vi "CloseNotifier.vi"(8 "entrée d'erreur":errorcluster caption="entrée d'erreur (pas d'erreur)", 11 "Notifiers":T1) -> (0 "error out":errorcluster)   [LabVIEW 2017, in "Notifier.lvlib"]
doc: "Ce VI permet la suppression de tous les notifiers à la fin de l'utilisation du centre d'usinage. Doit être modifier si un appareil a été ajouté ou supprimé."
uses:
  Notifier.lvlib
  Notifier.ctl
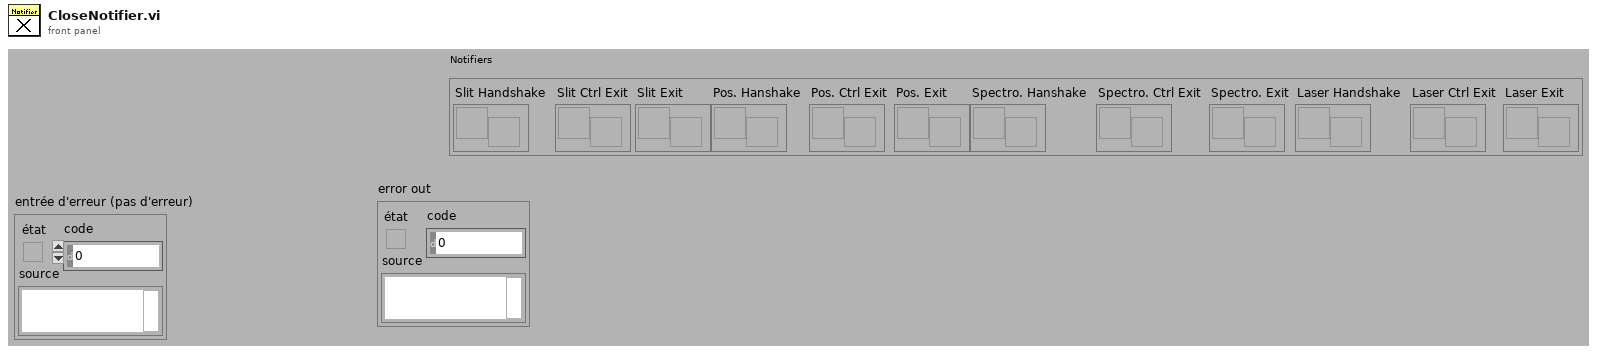
[diagram p1: front panel]
types:
  T1 = typedef "Notifier.lvlib/Notifier.ctl" = cluster{"Slit Handshake":refnum<notifier>, "Slit Ctrl Exit":refnum<notifier>, "Slit Exit":refnum<notifier>, "Pos. Hanshake":refnum<notifier>, "Pos. Ctrl Exit":refnum<notifier>, "Pos. Exit":refnum<notifier>, "Spectro. Hanshake":refnum<notifier>, "Spectro. Ctrl Exit":refnum<notifier>, "Spectro. Exit":refnum<notifier>, "Laser Handshake":refnum<notifier>, "Laser Ctrl Exit":refnum<notifier>, "Laser Exit":refnum<notifier>}
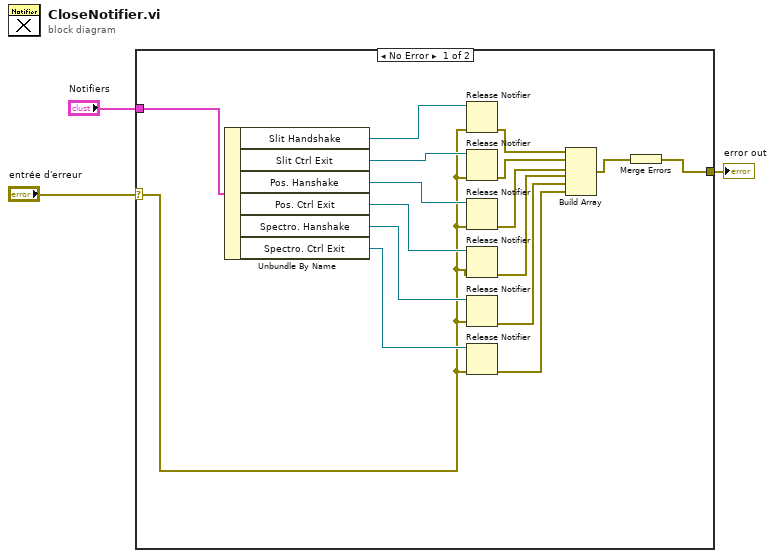
[diagram p0: block diagram]
diagram:
  n1 = case shown="No Error" "entrée d'erreur" {
    selector: "entrée d'erreur" -> [w4 w20]
    tunnel: "Notifiers" -> [w19 _]
    tunnel: [w11 w20] -> w1
    frame No Error {
      n2 = Unbundle By Name(w19) -> ("Slit Handshake"=w18:refnum<notifier>, "Slit Ctrl Exit"=w17:refnum<notifier>, "Pos. Hanshake"=w16:refnum<notifier>, "Pos. Ctrl Exit"=w10:refnum<notifier>, "Spectro. Hanshake"=w9:refnum<notifier>, "Spectro. Ctrl Exit"=w8:refnum<notifier>)
      n3 = Release Notifier(notifier=w18, error in (no error)=w4) -> (error out=w15:errorcluster)  [unwired: 1 in, 2 out]
      n4 = Release Notifier(notifier=w17, error in (no error)=w4) -> (error out=w14:errorcluster)  [unwired: 1 in, 2 out]
      n5 = Release Notifier(notifier=w16, error in (no error)=w4) -> (error out=w13:errorcluster)  [unwired: 1 in, 2 out]
      n6 = Release Notifier(notifier=w10, error in (no error)=w4) -> (error out=w7:errorcluster)  [unwired: 1 in, 2 out]
      n7 = Release Notifier(notifier=w9, error in (no error)=w4) -> (error out=w6:errorcluster)  [unwired: 1 in, 2 out]
      n8 = Release Notifier(notifier=w8, error in (no error)=w4) -> (error out=w5:errorcluster)  [unwired: 1 in, 2 out]
      n9 = Build Array(w15, w14, w13, w7, w6, w5) -> (w12:errorcluster[])
      n10 = Merge Errors(w12) -> (w11:errorcluster)
    }
    frame Error {
    }
  }
  "error out" <- w1
